vi "fromXML.vi"(8 "error in (no error)":errorcluster, 10 "xmlNode":refnum<class "xmlNode.lvclass">) -> (0 "error out":errorcluster, 3 "OutputConfiguration out":refnum<class "OutputConfiguration.lvclass">)   [LabVIEW 2009, in "Tools.lvlib" / "DatabaseHelpers.lvlib" / "OutputConfiguration.lvclass"]
uses:
  OutputConfiguration.lvclass
  xmlNode/xmlNode.lvclass
  OutputConfiguration.lvclass/OutputConfiguration.ctl
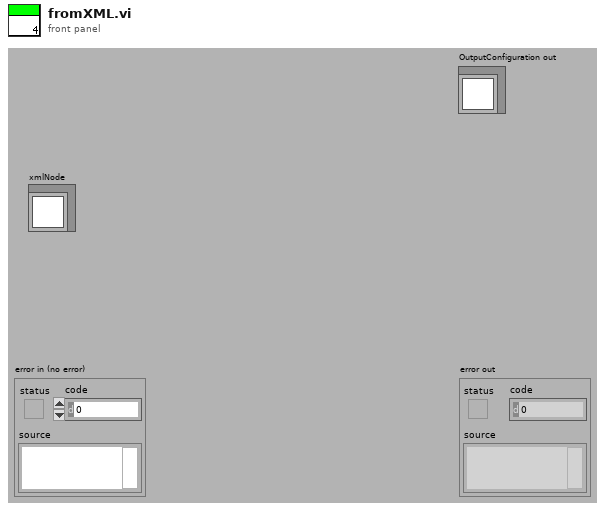
[diagram p1: front panel]
types:
  T1 = cluster{"stringValue":string, "stringValue":string}
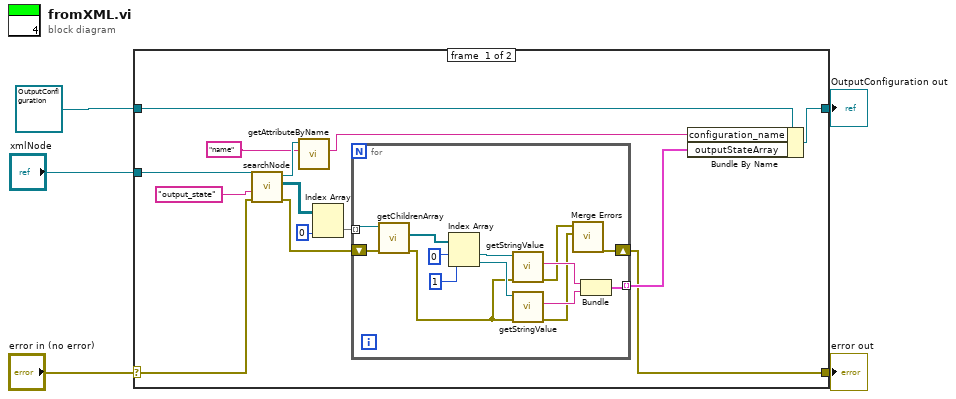
[diagram p0: block diagram]
diagram:
  n1 = case shown="No Error" "error in (no error)" {
    selector: "error in (no error)" -> [w11 w35]
    tunnel: [w9 w35] -> w4
    tunnel: [w12 w34] -> w3
    tunnel: refnum<class "OutputConfiguration.lvclass"> refnum ("OutputConfiguration in") -> [w13 w34]
    tunnel: "xmlNode" -> [w19 _]
    frame #0 {
      n2 = call-dynamic "searchNode.vi"("error in (no error)"=w11, "searchElementName"="output_state", "xmlNode in"=w19) -> ("error out"=w10:errorcluster, "arrayXmlNodes"=w17:refnum<class "xmlNode.lvclass">[][], "xmlNode out"=w8:refnum<class "xmlNode.lvclass">)  [unwired: 6 in]
      n3 = call-dynamic "getAttributeByName.vi"("AttributeName"="name", "xmlNode in"=w8) -> ("attribute string"=w6:string)  [unwired: 7 in, 2 out]
      n4 = Index Array(array=w17, index (col)=0) -> (element=w15:refnum<class "xmlNode.lvclass">[])  [unwired: 1 in]
      n5 = for {
        tunnel: w15 -> [w33] mode=indexing
        tunnel: [w25] -> w14 mode=indexing
        shift-right: [w20] -> w9
        shift-left: w10 -> [w24]
        n6 = call-dynamic "getChildrenArray.vi"("error in (no error)"=w24, "xmlNode.lvclass in"=w33) -> ("error out"=w23:errorcluster, "Children"=w32:refnum<class "xmlNode.lvclass">[])  [unwired: 7 in, 1 out]
        n7 = Index Array(array=w32, index #1=0, index #2=1) -> (element #1=w29:refnum<class "xmlNode.lvclass">, element #2=w28:refnum<class "xmlNode.lvclass">)
        n8 = call-dynamic "getStringValue.vi"("error in (no error)"=w23, "xmlNode.lvclass in"=w29) -> ("error out"=w22:errorcluster, "stringValue"=w27:string)  [unwired: 7 in, 1 out]
        n9 = call-dynamic "getStringValue.vi"("error in (no error)"=w23, "xmlNode.lvclass in"=w28) -> ("error out"=w21:errorcluster, "stringValue"=w26:string)  [unwired: 7 in, 1 out]
        n10 = call <vilib>:"Merge Errors.vi"("error in 2 (no error)"=w21, "error in 1 (no error)"=w22) -> ("error out"=w20:errorcluster)  [unwired: 5 in]
        n11 = Bundle("stringValue"=w27, "stringValue"=w26) -> (w25:T1)  [unwired: 1 in]
      }
      n12 = Bundle By Name(cluster=w13, "configuration_name"=w6, "outputStateArray"=w14) -> (w12:refnum<class "OutputConfiguration.lvclass">)
    }
    frame #1 {
    }
  }
  "error out" <- w4
  "OutputConfiguration out" <- w3
